vi "OscRead-Com-Exec.vi"(5 "ControlQueue":refnum<queue>, 6 "Timeout (10000 ms)":u32=10000, 8 "error in (no error)":errorcluster, 9 "data":variant, 10 "Multiple":bool=TRUE, 11 "Oscilloscope in":refnum<class "Oscilloscope.lvclass">) -> (0 "error out":errorcluster, 2 "Waveform Data OUT":waveform(dbl)[](graph), 3 "Oscilloscope out":refnum<class "Oscilloscope.lvclass">)   [LabVIEW 2019, in "Oscilloscope.lvclass"]
uses:
  Oscilloscope.lvclass
  C:/Users/elysium/Documents/dev/TRANCON/Classes/GeneralFunctionality/GeneralFunctionality.lvclass
  GeneralFunctionality/GeneralFunctionality.lvclass/GeneralFunctionality.ctl
  dependecies/ControlsVIs/Clusters-def/SERVER-Commands.ctl
  dependecies/ControlsVIs/Clusters-def/OSc-Reply-Read.ctl
  dependecies/ControlsVIs/Clusters-def/OSc-Demand-Read.ctl
  Oscilloscope.lvclass/Oscilloscope.ctl
  dependecies/ControlsVIs/Clusters-def/Message types.ctl
  Message/Message.lvclass
  TELEDINE_LECROY/LeCroy Wave Series/LeCroy Wave Series.lvlib
  Control/Control-Server/Control-Server.lvclass
  GeneralFunctionality/GeneralFunctionality.lvclass
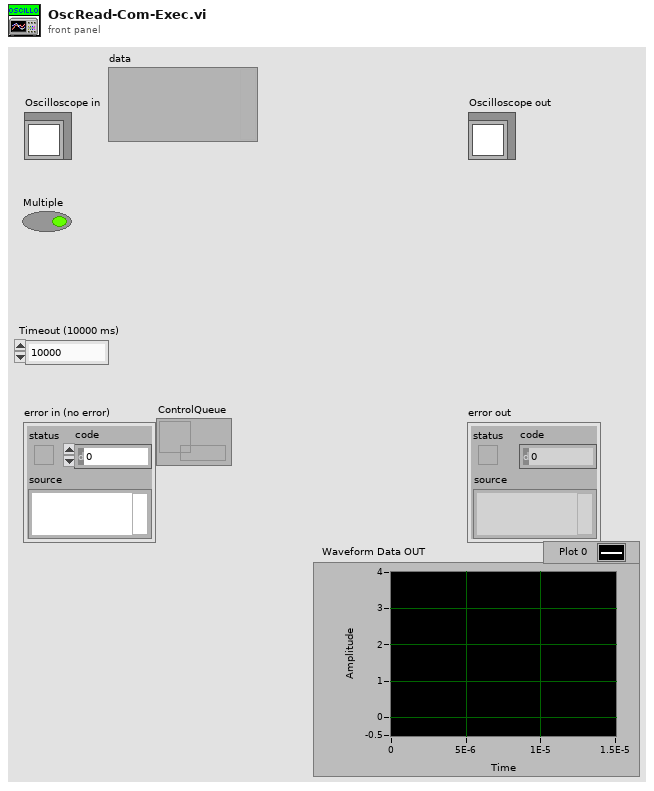
[diagram p1: front panel]
types:
  T1 = typedef "Oscilloscope.lvclass/OSc-Reply-Read.ctl" = cluster{"Data":waveform(dbl)[], "Channels":u16[], "error":errorcluster}
  T2 = typedef "Control-Server.lvclass/SERVER-Commands.ctl" = string
  T3 = typedef "Message types.ctl" = string
  T4 = typedef "Oscilloscope.lvclass/OSc-Demand-Read.ctl" = cluster{"ON/OFF":bool, "Channels":u16[]}
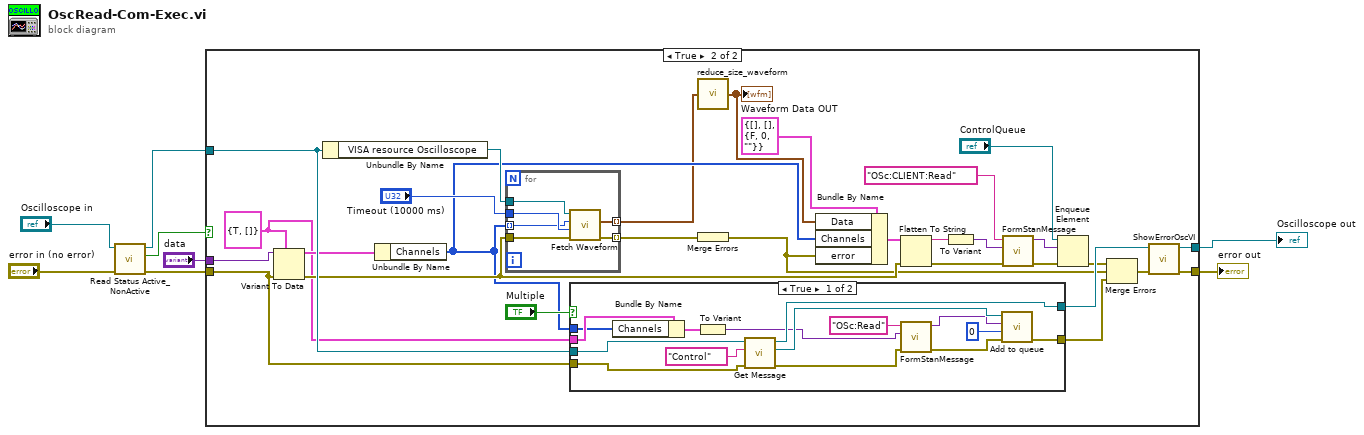
[diagram p0: block diagram]
diagram:
  n1 = call "Read Status Active_NonActive.vi"("error in (no error)"="error in (no error)", "GeneralFunctionality in"="Oscilloscope in") -> ("error out"=w2:errorcluster, "Status Active/NonActive"=w3:bool, "GeneralFunctionality out"=w4:refnum<class "Oscilloscope.lvclass">)  [unwired: 7 in]
  n2 = case shown="True" w3 {
    tunnel: [w10 w35] -> w8
    tunnel: [w9 w36] -> w7
    tunnel: w4 -> [w10 w33]
    tunnel: w2 -> [w9 w19]
    tunnel: "data" -> [_ w16]
    frame False {
    }
    frame True {
      w17 = T4 {"ON/OFF"=TRUE, "Channels"=[]}
      n3 = Variant To Data(error in=w19, type=w17, Variant=w16) -> (data=w20:T4, error out=w18:errorcluster)
      n4 = Unbundle By Name(w33) -> ("VISA resource Oscilloscope"=w32:refnum<visa-resource-name>)
      n5 = Unbundle By Name(w20) -> ("Channels"=w13:u16[])
      n6 = for {
        tunnel: w32 -> [w45]
        tunnel: "Timeout (10000 ms)" -> [w44]
        tunnel: [w40] -> w12 mode=indexing
        tunnel: w18 -> [w42]
        tunnel: [w43] -> w15 mode=indexing
        tunnel: w13 -> [w41] mode=indexing
        n7 = call "Fetch Waveform.vi"("error in (no error)"=w42, "Timeout (10000 ms)"=w44, "Source (0: Channel 1)"=w41, "VISA resource name"=w45) -> ("error out"=w43:errorcluster, "Waveform Graph"=w40:waveform(dbl))  [unwired: 5 in, 1 out]
      }
      n8 = case shown="True" "Multiple" {
        tunnel: [w60 w61] -> w39
        tunnel: [w56 w62] -> w38
        tunnel: w33 -> [w54 w61]
        tunnel: w19 -> [w53 w62]
        tunnel: w17 -> [w47 _]
        tunnel: w13 -> [w46 _]
        frame True {
          n9 = Bundle By Name(cluster=w47, "Channels"=w46) -> (w55:T4)
          n10 = To Variant(anything=w55) -> (Variant=w51:variant)
          n11 = call "Get Message.vi"("error in (no error)"=w53, "Message type"=T3 "Control", "GeneralFunctionality en entrée"=w54) -> ("error out"=w50:errorcluster, "Message.lvclass"=w59:refnum<class "Message.lvclass">, "GeneralFunctionality en sortie"=w60:refnum<class "Oscilloscope.lvclass">)  [unwired: 6 in]
          n12 = call "FormStanMessage.vi"("error in"=w50, "data"=w51, "Command"="OSc:Read" ("command")) -> ("error out"=w49:errorcluster, "message"=w48:variant)  [unwired: 7 in]
          n13 = call "Add to queue.vi"("error in (no error)"=w49, "timeout in ms (-1)"=0, "Data"=w48, "Message in"=w59) -> ("error out"=w56:errorcluster)  [unwired: 6 in, 1 out]
        }
        frame False {
        }
      }
      n14 = call "reduce_size_waveform.vi"("Waveform Data IN"=w12) -> ("Waveform Data OUT"=w11:waveform(dbl)[])
      "Waveform Data OUT" <- w11
      n15 = Merge Errors(w15) -> (w14:errorcluster)
      n16 = Bundle By Name(cluster=T1 {"Data"=[], "Channels"=[], "error"={"status"=FALSE, "code"=0, "source"=""}}, "Data"=w11, "Channels"=w13, "error"=w14) -> (w27:T1)
      n17 = Flatten To String(anything=w27, error in (no error)=w18) -> (data string=w30:string, error out=w25:errorcluster)  [unwired: 2 in, 1 out]
      n18 = To Variant(anything=w30) -> (Variant=w21:variant)
      n19 = call "FormStanMessage.vi"("error in"=w25, "data"=w21, "Command"=T2 "OSc:CLIENT:Read" ("Commands")) -> ("error out"=w24:errorcluster, "message"=w23:variant)  [unwired: 7 in]
      n20 = Enqueue Element(queue="ControlQueue", element=w23, error in (no error)=w24) -> (error out=w26:errorcluster)  [unwired: 1 in, 2 out]
      n21 = Merge Errors(w26, w14, w38) -> (w37:errorcluster)
      n22 = call "ShowErrorOscVI.vi"("error in (no error)"=w37, "Oscilloscope in"=w39) -> ("error out"=w36:errorcluster, "Oscilloscope out"=w35:refnum<class "Oscilloscope.lvclass">)  [unwired: 8 in]
    }
  }
  "error out" <- w7
  "Oscilloscope out" <- w8
